vi "_AllThingsEdgertronic.vi"() -> ()   [LabVIEW 2015]
panel:
  in  "Setup":T1={"URL"="130.64.16.195", "remote port"=80, "mode (standard)"=enum."Standard"}
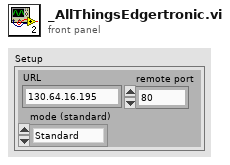
[diagram p1: front panel]
types:
  T1 = cluster{"URL":string, "remote port":u16, "mode (standard)":enum16{"Standard", "Buffered", "CRLF", "Immediate"}}
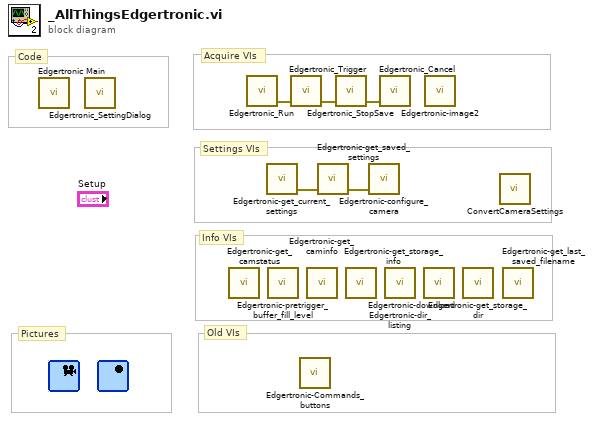
[diagram p0: block diagram]
diagram:
  # "Code"
  # "Pictures"
  # "Acquire VIs"
  # "Settings VIs"
  # "Info VIs"
  # "Old VIs"
  n1 = call "Edgertronic Main.vi"() -> ()  [unwired: 12 in]
  n2 = call "Edgertronic_SettingDialog.vi"() -> ()  [unwired: 3 in, 1 out]
  n3 = call "Edgertronic-get_camstatus.vi"() -> ()  [unwired: 3 in, 3 out]
  n4 = call "Edgertronic_Run.vi"() -> ("error out"=w1:errorcluster)  [unwired: 5 in]
  n5 = call "Edgertronic-get_current_settings.vi"() -> ("error out"=w5:errorcluster)  [unwired: 4 in, 1 out]
  n6 = call "Edgertronic-pretrigger_buffer_fill_level.vi"() -> ()  [unwired: 3 in, 3 out]
  n7 = call "Edgertronic_Trigger.vi"("error in (no error)"=w1) -> ("error out"=w3:errorcluster)  [unwired: 4 in]
  n8 = call "Edgertronic-Commands_buttons.vi"() -> ()  [unwired: 4 in, 2 out]
  n9 = call "Edgertronic-get_caminfo.vi"() -> ()  [unwired: 4 in, 2 out]
  n10 = call "Edgertronic-get_saved_settings.vi"("error in (no error)"=w5) -> ("error out"=w4:errorcluster)  [unwired: 3 in, 1 out]
  n11 = call "Edgertronic_StopSave.vi"("error in (no error)"=w3) -> ("error out"=w2:errorcluster)  [unwired: 4 in]
  n12 = call "Edgertronic-get_storage_info.vi"() -> ()  [unwired: 3 in, 3 out]
  n13 = call "Edgertronic-configure_camera.vi"("error in (no error)"=w4) -> ()  [unwired: 3 in, 2 out]
  n14 = call "Edgertronic_Cancel.vi"("error in (no error)"=w2) -> ()  [unwired: 4 in, 1 out]
  n15 = call "Edgertronic-dir_listing.vi"() -> ()  [unwired: 3 in, 3 out]
  n16 = call "Edgertronic-download.vi"() -> ()  [unwired: 4 in, 2 out]
  n17 = call "Edgertronic-image2.vi"() -> ()  [unwired: 3 in, 3 out]
  n18 = call "Edgertronic-get_storage_dir.vi"() -> ()  [unwired: 4 in, 2 out]
  n19 = call "ConvertCameraSettings.vi"() -> ()  [unwired: 1 in, 1 out]
  n20 = call "Edgertronic-get_last_saved_filename.vi"() -> ()  [unwired: 4 in, 2 out]
